vi "Add SR Popup.vi"(8 "error in":errorcluster) -> (0 "error out":errorcluster, 2 "New SR?":bool, 3 "SR array out":i32[](array[numeric]))   [LabVIEW 2018]
uses:
  <vilib>/Utility/miscctls.llb/LVPointTypeDef.ctl
panel:
  in  "Close":bool
  in  "Add SR":bool
  in  "SR to Add":string
  # "Enter SR number(s) seperated by commas\n and press \"Add SR\" to add it to the list"
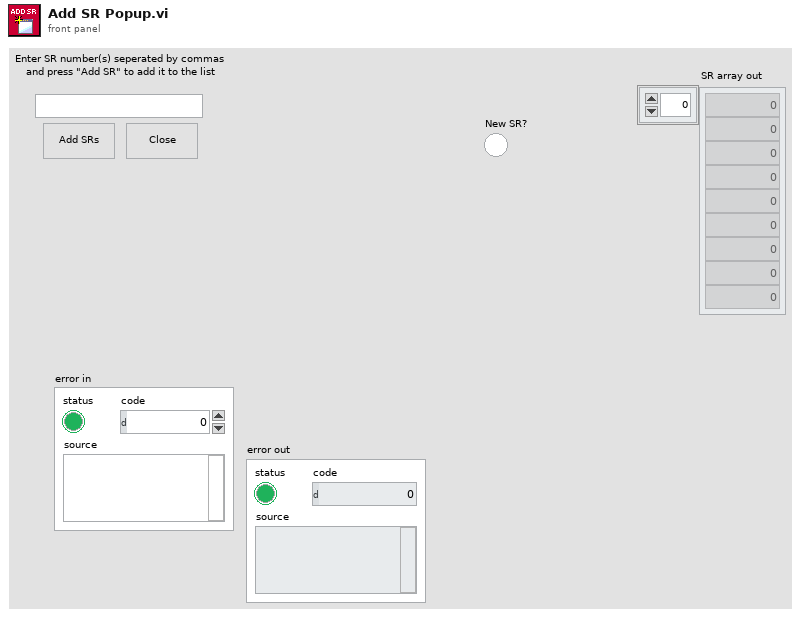
[diagram p1: front panel]
types:
  T1 = typedef "LVPointTypeDef.ctl" = cluster{"Horizontal":i16, "Vertical":i16}
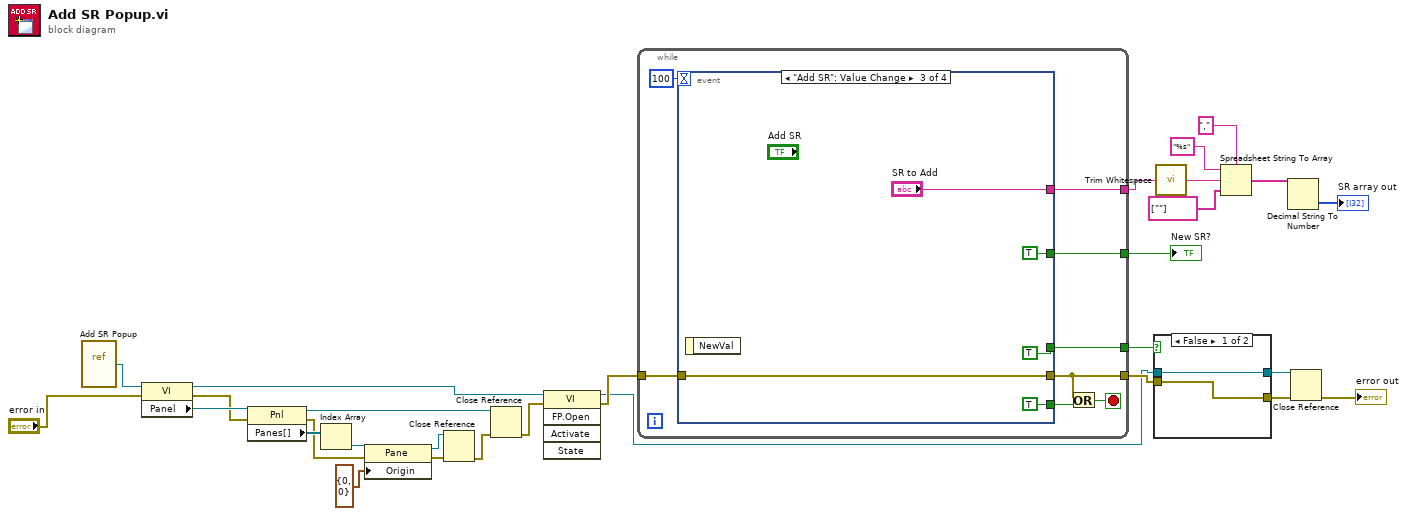
[diagram p0: block diagram]
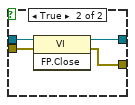
[diagram p2: hidden frame]
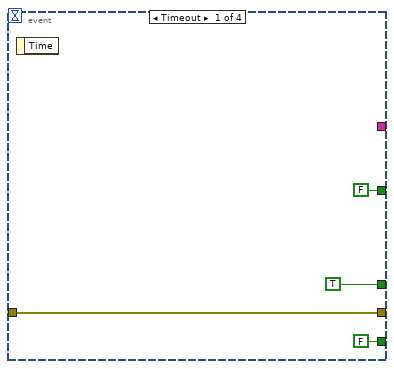
[diagram p3: hidden frame]
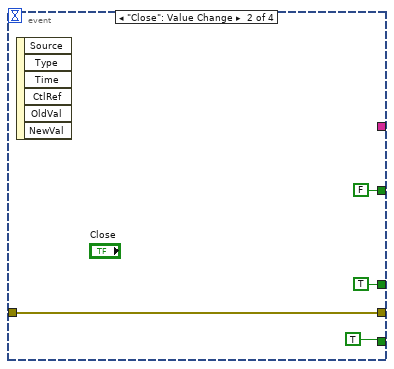
[diagram p4: hidden frame]
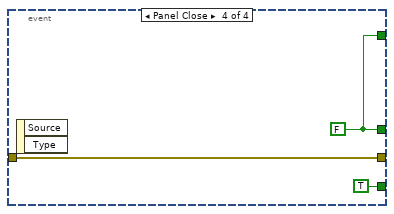
[diagram p5: hidden frame]
diagram:
  n1 = vi-ref "Add SR Popup.vi"() -> (w29:refnum<vi>)
  n2 = property class="VI"(reference=w29, error in="error in") -> (reference out=w12:refnum<vi>, error out=w19:errorcluster, "Panel"=w20:refnum<vi>)
  n3 = property class="Pnl"(reference=w20, error in=w19) -> (reference out=w21:refnum<vi>, error out=w26:errorcluster, "Panes[]"=w28:refnum<vi>[])
  n4 = Index Array(array=w28) -> (element=w27:refnum<vi>)  [unwired: 1 in]
  n5 = property class="Pane"(reference=w27, error in=w26, "Origin"=T1 {"Horizontal"=0, "Vertical"=0}) -> (reference out=w24:refnum<vi>, error out=w23:errorcluster)
  n6 = Close Reference(reference=w24, error in (no error)=w23) -> (error out=w22:errorcluster)
  n7 = Close Reference(reference=w21, error in (no error)=w22) -> (error out=w11:errorcluster)
  n8 = invoke class="VI" method="FP.Open"(reference=w12, error in=w11) -> (reference out=w13:refnum<vi>, error out=w18:errorcluster)  [unwired: 3 in, 3 out]
  n9 = while {
    tunnel: w18 -> [w35]
    tunnel: [w33] -> w17
    tunnel: [w36] -> w1
    tunnel: [w31] -> w9
    tunnel: [w30] -> w7
    stop <- w34 stop-if-true
    n10 = event shown="[2] \"Add SR\": Value Change" {
      selector: _ -> [_ _ _ _]
      dyn-events: _ -> [_ _ _ _]
      timeout: 100 -> [_ _ _ _]
      tunnel: w35 -> [w40 w43 w50 w53]
      tunnel: [w40 w43 w50 w53] -> w33
      tunnel: [TRUE TRUE TRUE w51] -> w36
      tunnel: [FALSE TRUE TRUE TRUE] -> w32
      tunnel: [FALSE FALSE TRUE w51] -> w31
      tunnel: [_ _ "SR to Add" _] -> w30
      event Timeout {
        n11 = event-data() -> ()  [unwired: 1 in, 1 out]
      }
      event "Close": Value Change {
        n12 = event-data() -> ()  [unwired: 1 in, 6 out]
      }
      event "Add SR": Value Change {
        n13 = event-data() -> ()  [unwired: 1 in, 1 out]
      }
      event Panel Close {
        w51 = FALSE
        n14 = event-data() -> ()  [unwired: 1 in, 2 out]
      }
    }
    n15 = Or(x=w33, y=w32) -> (x .or. y?=w34:bool)
  }
  "New SR?" <- w9
  n16 = case shown="False" w1 {
    tunnel: w13 -> [w55 w59]
    tunnel: w17 -> [w54 w58]
    tunnel: [w55 w57] -> w16
    tunnel: [w54 w56] -> w15
    frame False {
    }
    frame True {
      n17 = invoke class="VI" method="FP.Close"(reference=w59, error in=w58) -> (reference out=w57:refnum<vi>, error out=w56:errorcluster)  [unwired: 1 in, 1 out]
    }
  }
  n18 = call <vilib>:"Trim Whitespace.vi"("string"=w7) -> ("trimmed string"=w6:string)  [unwired: 1 in]
  n19 = Spreadsheet String To Array(delimiter (Tab)=",", format string="%s", spreadsheet string=w6, array type (2D Dbl)=string[] [""]) -> (array=w3:string[])
  n20 = Decimal String To Number(string=w3) -> (number=→"SR array out":i32[])  [unwired: 2 in, 1 out]
  n21 = Close Reference(reference=w16, error in (no error)=w15) -> (error out=→"error out":errorcluster)
